vi "CloseModuleManager.vi"(8 "error in (no error)":errorcluster, 11 "Sensor Engine Datas in":T1[](array[typedef]) {"MM Frames"."payload" format="%x"; "MM Frames"."timestamp" format="%<%.7X\n%x>T"; "MM Frames"."type" items=["FlexRay Data"=32, "FlexRay Null"=33, "FlexRay Symbol"=34, "Log Trigger"=225, "Start Trigger"=226]; "MM Frames"."cycle count" max=63 step=1}) -> (0 "error out":errorcluster, 3 "Sensor Engine Datas out":T1[](array[typedef]) {"MM Frames"."payload" format="%x"; "MM Frames"."timestamp" format="%<%.7X\n%x>T"; "MM Frames"."type" items=["FlexRay Data"=32, "FlexRay Null"=33, "FlexRay Symbol"=34, "Log Trigger"=225, "Start Trigger"=226]; "MM Frames"."cycle count" max=63 step=1})   [LabVIEW 2018, in "MM.lvlib"]
uses:
  MM.lvlib
  Sensor Engine Data.ctl
  Shared/Protocol.ctl
  Shared/Sensor Name.ctl
  <vilib>/xnet/xnet.llb/XNET Frame FlexRay.ctl
  <vilib>/xnet/xnet.llb/XNET Frame Type FlexRay.ctl
  Shared/Vires VTD Shared.lvlib
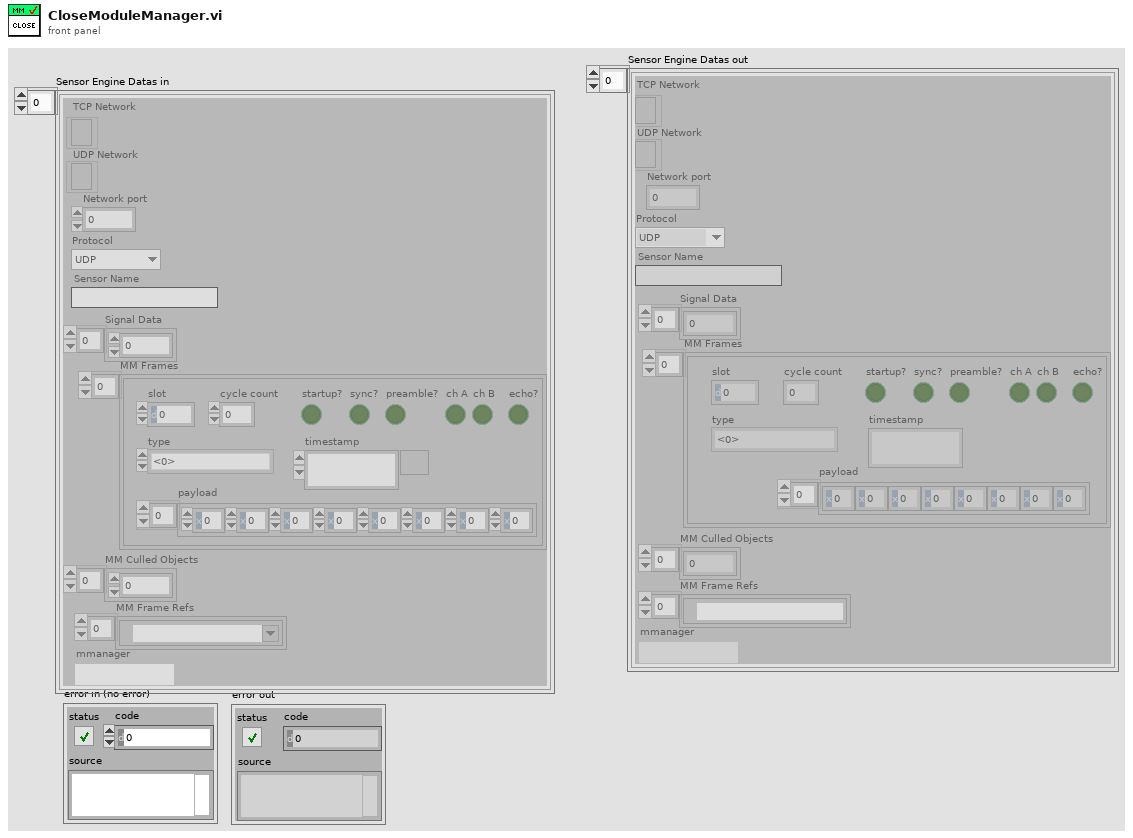
[diagram p1: front panel]
types:
  T1 = typedef "MM.lvlib/Sensor Engine Data.ctl" = cluster{"TCP Network":refnum<k5>, "UDP Network":refnum<k16>, "Network port":i32, "Protocol":T2, "Sensor Name":T3, "Signal Data":dbl[], "MM Frames":T4[], "MM Culled Objects":i32[], "MM Frame Refs":refnum<k21>[], "mmanager":path}
  T2 = typedef "Vires VTD Shared.lvlib/Protocol.ctl" = enum16{"UDP", "TCP"}
  T3 = typedef "Vires VTD Shared.lvlib/Sensor Name.ctl" = string
  T4 = typedef "XNET Frame FlexRay.ctl" = cluster{"timestamp":timestamp, "payload":u8[], "slot":u16, "type":T5, "cycle count":u8, "startup?":bool, "sync?":bool, "preamble?":bool, "ch A":bool, "ch B":bool, "echo?":bool}
  T5 = typedef "XNET Frame Type FlexRay.ctl" = u8
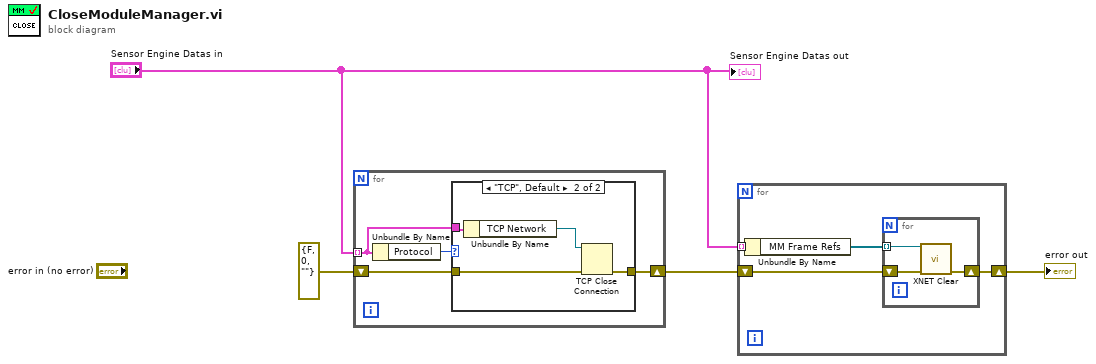
[diagram p0: block diagram]
diagram:
  n1 = for {
    shift-right: [w7] -> w4
    shift-left: errorcluster {"status"=FALSE, "code"=0, "source"=""} ("error out") -> [w8]
    tunnel: "Sensor Engine Datas in" -> [w5] mode=indexing
    n2 = Unbundle By Name(w5) -> ("Protocol"=w6:T2)
    n3 = case shown="\"TCP\", Default" w6 {
      tunnel: w8 -> [w9 w13]
      tunnel: [w9 w12] -> w7
      tunnel: w5 -> [_ w11]
      frame "UDP" {
      }
      frame "TCP", Default {
        n4 = Unbundle By Name(w11) -> ("TCP Network"=w10:refnum<k5>)
        n5 = TCP Close Connection(connection ID=w10, error in (no error)=w13) -> (error out=w12:errorcluster)  [unwired: 1 in, 1 out]
      }
    }
  }
  n6 = for {
    shift-right: [w16] -> w3
    shift-left: w4 -> [w17]
    tunnel: "Sensor Engine Datas in" -> [w15] mode=indexing
    n7 = Unbundle By Name(w15) -> ("MM Frame Refs"=w14:refnum<k21>[])
    n8 = for {
      shift-right: [w19] -> w16
      shift-left: w17 -> [w20]
      tunnel: w14 -> [w18] mode=indexing
      n9 = call <vilib>:"XNET Clear.vi"("session in"=w18, "error in (no error)"=w20) -> ("error out"=w19:errorcluster)  [unwired: 13 in]
    }
  }
  "error out" <- w3
  "Sensor Engine Datas out" <- "Sensor Engine Datas in"
